vi "File.Convert String to CSV Item.vi"(11 "String":string) -> (3 "String Out":string)   [LabVIEW 2024, in "EQMF.lvlib" / "File Utils.lvlib"]
uses:
  File Utils.lvlib
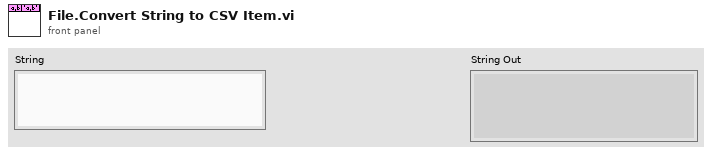
[diagram p1: front panel]
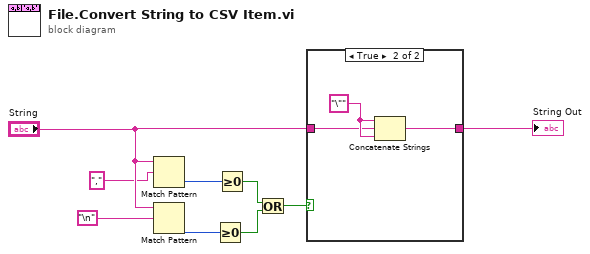
[diagram p0: block diagram]
diagram:
  n1 = Match Pattern(string="String", regular expression=",") -> (offset past match=w8:i32)  [unwired: 1 in, 3 out]
  n2 = Match Pattern(string="String", regular expression="\n") -> (offset past match=w7:i32)  [unwired: 1 in, 3 out]
  n3 = Greater Or Equal To 0?(x=w7) -> (x >= 0?=w5:bool)
  n4 = Greater Or Equal To 0?(x=w8) -> (x >= 0?=w6:bool)
  n5 = Or(x=w6, y=w5) -> (x .or. y?=w4:bool)
  n6 = case shown="True" w4 {
    tunnel: "String" -> [w10 w12]
    tunnel: [w10 w11] -> w2
    frame False {
    }
    frame True {
      w13 = "\""
      n7 = Concatenate Strings(w13, w12, w13) -> (w11:string)
    }
  }
  "String Out" <- w2
